vi "Inicio.vi"(8 "error in (no error)":errorcluster, 11 "Data":variant) -> (0 "error out":errorcluster)   [LabVIEW 2019, in "Prueba05.lvclass"]
uses:
  Prueba05.lvclass
  Queues/Private Controls/Prueba5 Estados.ctl
  Queues/Private Controls/Prueba5 Data Cluster.ctl
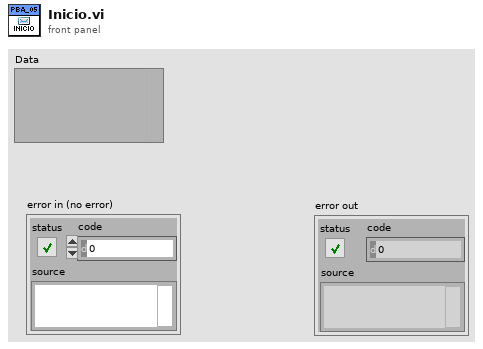
[diagram p1: front panel]
types:
  T1 = typedef "Prueba05.lvclass/Prueba5 Data Cluster.ctl" = cluster{"Estados":T2, "Data":variant}
  T2 = typedef "Prueba05.lvclass/Prueba5 Estados.ctl" = enum16{"inicio", "salir"}
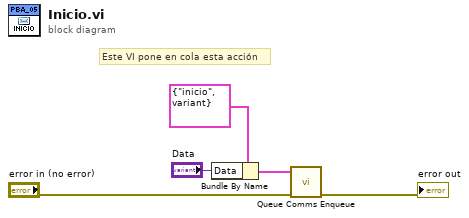
[diagram p0: block diagram]
diagram:
  # "Este VI pone en cola esta acción"
  n1 = Bundle By Name(cluster=T1 {"Estados"=enum."inicio", "Data"=variant} ("Element"), "Data"="Data") -> (w2:T1)
  n2 = call "Queue Comms Enqueue.vi"("error in (no error)"="error in (no error)", "Element"=w2) -> ("error out"=→"error out":errorcluster)  [unwired: 8 in, 1 out]
